vi "SetPicture.vi"(0 "reference":refnum<class "Graphics.lvclass">, 1 "picture":picture, 5 "error in (no error)":errorcluster) -> (14 "reference out":refnum<class "Graphics.lvclass">, 19 "error out":errorcluster)   [LabVIEW 2016, in "Graphics.lvclass"]
uses:
  <resource>/Framework/Providers/Open_GDS/UML/Graphics_class/Graphics.lvclass
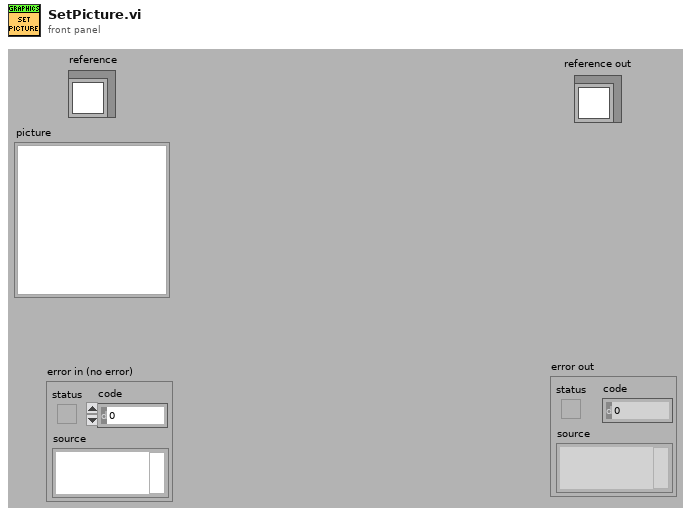
[diagram p1: front panel]
types:
  T1 = typedef "Graphics.lvclass/ObjectAttributes.ctl" = cluster{"drawColor":u32, "backgroundColor":u32, "font":T2, "fontType":T3, "picture":picture, "stroke":T4, "scaleX":dbl, "scaleY":dbl, "screenRef":refnum<vi>, "offsetX":dbl, "offsetY":dbl}
  T2 = typedef "Graphics.lvclass/FontType.ctl" = cluster{"Font Name:":string, "Size":i16, "Strikeout?":bool, "Italic?":bool, "Underline?":bool, "Outline?":bool, "Shadow?":bool, "Bold?":bool}
  T3 = typedef "Graphics.lvclass/LvFontType.ctl" = enum16{"User-specified Font", "Application Font", "System Font", "Dialog Font"}
  T4 = typedef "Graphics.lvclass/StrokeType.ctl" = enum16{"USE_DEFAULT", "SOLID", "DOTTED"}
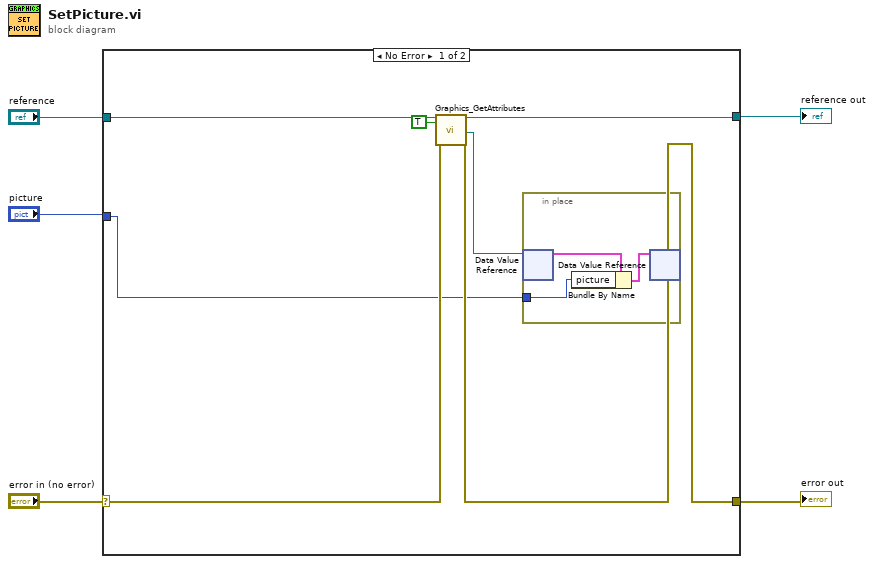
[diagram p0: block diagram]
diagram:
  n1 = case shown="No Error" "error in (no error)" {
    selector: "error in (no error)" -> [w12 w16]
    tunnel: "reference" -> [w11 w17]
    tunnel: [w10 w16] -> w3
    tunnel: [w9 w17] -> w2
    tunnel: "picture" -> [w6 _]
    frame No Error {
      n2 = call <resource>:"Graphics_GetAttributes.vi"("reference in"=w11, "OnlyGetDvrReference(False)"=TRUE, "error in (no error)"=w12) -> ("reference out"=w9:refnum<class "Graphics.lvclass">, "DataRef"=w7:refnum<data-value>, "error out"=w10:errorcluster)  [unwired: 13 in, 1 out]
      n3 = in-place {
        in-place-border: w6 -> [w14]
        n4 = in-place-dvr #1(w7) -> (w15:T1)  [unwired: 1 out]
        n5 = Bundle By Name(cluster=w15, "picture"=w14) -> (w13:T1)
        n6 = in-place-dvr #1(w13) -> ()  [unwired: 2 out]
      }
    }
    frame Error {
    }
  }
  "reference out" <- w2
  "error out" <- w3
